vi "Init Actor.vi"() -> (3 "Actor":refnum<class "Actor.lvclass">)   [LabVIEW 2020, in "jettl.lvlib" / "BaseActor.lvlib"]
uses:
  BaseActor.lvlib
  Base Actor/Base Actor.lvclass
  Actor/Actor.lvclass
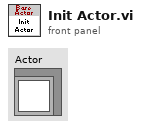
[diagram p1: front panel]
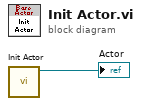
[diagram p0: block diagram]
diagram:
  n1 = call "Init Actor.vi"() -> ("Base Actor out"=→"Actor":refnum<class "Base Actor.lvclass">)  [unwired: 11 in]
